vi "Show Front Panel.vi"(8 "error in (no error)":errorcluster, 11 "Receiver in":refnum<class "Receiver.lvclass">) -> (0 "error out":errorcluster, 3 "Receiver out":refnum<class "Receiver.lvclass">)   [LabVIEW 2013, in "Receiver.lvlib" / "Receiver.lvclass"]
uses:
  Receiver.lvclass
  Receiver.lvclass/Receiver.ctl
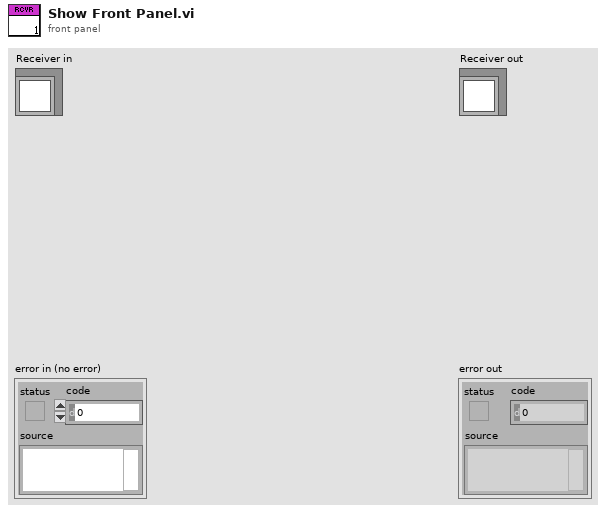
[diagram p1: front panel]
types:
  T1 = enum32{"Invalid", "Standard", "Closed", "Hidden", "Minimized", "Maximized"}
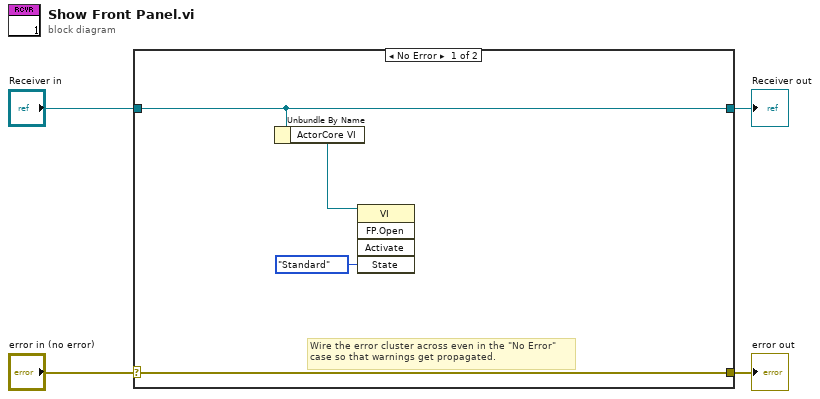
[diagram p0: block diagram]
diagram:
  n1 = case shown="No Error" "error in (no error)" {
    selector: "error in (no error)" -> [w8 w10]
    tunnel: [w8 w10] -> w3
    tunnel: [w6 w9] -> w1
    tunnel: "Receiver in" -> [w6 w9]
    frame No Error {
      # "Wire the error cluster across even in the \"No Error\"\ncase so that warnings get propagated."
      n2 = Unbundle By Name(w6) -> ("ActorCore VI"=w5:refnum<vi>)
      n3 = invoke class="VI" method="FP.Open"(reference=w5, "State"=T1."Standard") -> ()  [unwired: 3 in, 5 out]
    }
    frame Error {
    }
  }
  "error out" <- w3
  "Receiver out" <- w1
